vi "Read Dwell Time.vi"(8 "error in (no error)":errorcluster, 11 "LCD Reader.lvclass in":refnum<class "LCD Reader.lvclass">) -> (0 "error out":errorcluster, 1 "Most Specific Classname":string, 2 "Dwell Time":dbl[unit], 3 "LCD Reader.lvclass out":refnum<class "LCD Reader.lvclass">)   [LabVIEW 2017, in "LCD Reader.lvclass"]
doc: "Return the pre-set dwell time inside this Reader instance."
uses:
  LCD Reader.lvclass
  LCD Reader.lvclass/LCD Reader.ctl
  Reader/Reader.lvclass
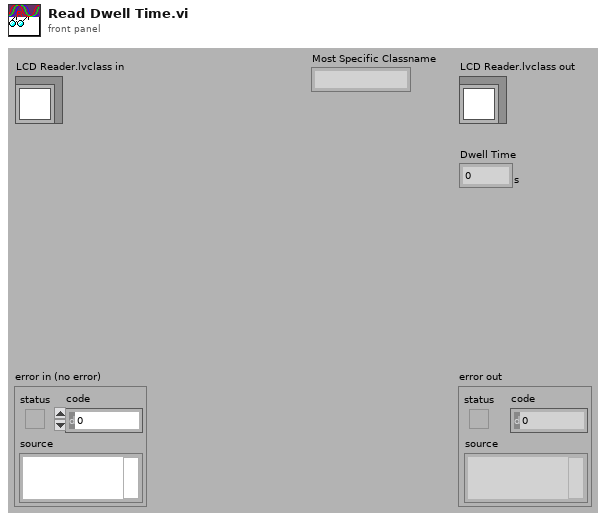
[diagram p1: front panel]
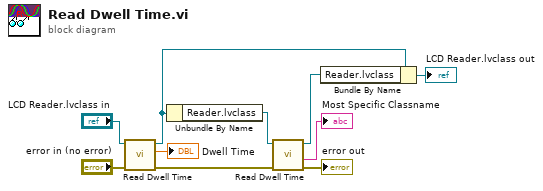
[diagram p0: block diagram]
diagram:
  n1 = call-parent "Read Dwell Time.vi"("error in (no error)"="error in (no error)", "Reader.lvclass in"="LCD Reader.lvclass in") -> ("error out"=w2:errorcluster, "Dwell Time"=→"Dwell Time":dbl[unit], "Reader.lvclass out"=w7:refnum<class "LCD Reader.lvclass">)  [unwired: 6 in, 1 out]
  n2 = Unbundle By Name(w7) -> ("Reader.lvclass"=w6:refnum<class "Reader.lvclass">)
  n3 = call-dynamic "Read Dwell Time.vi"("error in (no error)"=w2, "Reader.lvclass in"=w6) -> ("error out"=→"error out":errorcluster, "Most Specific Classname"=→"Most Specific Classname":string, "Reader.lvclass out"=w3:refnum<class "Reader.lvclass">)  [unwired: 6 in, 1 out]
  n4 = Bundle By Name(cluster=w7, "Reader.lvclass"=w3) -> (→"LCD Reader.lvclass out":refnum<class "LCD Reader.lvclass">)
